vi "Open COM Port.vi"(8 "error in (no error)":errorcluster) -> (0 "error out":errorcluster, 3 "VISA Refnum out":refnum<visa-resource-name>)   [LabVIEW 2017]
uses:
  <vilib>/Instr/_visa.llb/VISA Configure Serial Port (Instr).vi
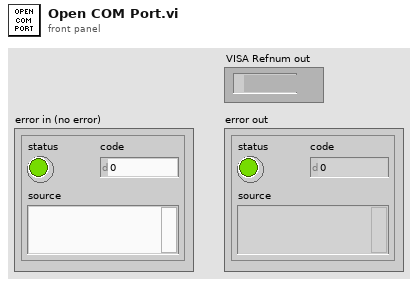
[diagram p1: front panel]
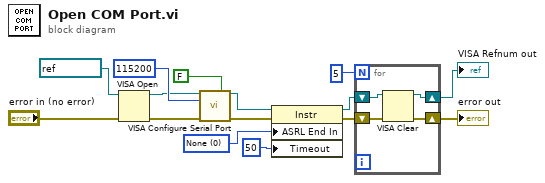
[diagram p0: block diagram]
diagram:
  w7 = u16 0 items=["None", "Last Bit", "TermChar"] ("Serial Settings:End Mode for Reads")
  n1 = VISA Open(error in (no error)="error in (no error)", VISA resource name=refnum<visa-resource-name> "COM2") -> (VISA resource name=w3:refnum<visa-resource-name>, error out=w2:errorcluster)  [unwired: 3 in]
  n2 = call-poly "VISA Configure Serial Port"("VISA resource name"=w3, "Enable Termination\nChar (T)"=FALSE ("Enable Termination\nChar (T)"), "baud rate (9600)"=u32 115200, "error in (no error)"=w2) -> ("VISA resource name out"=w6:refnum<visa-resource-name>, "error out"=w8:errorcluster)  [unwired: 10 in]
  n3 = property class="Instr"(reference=w6, error in=w8, "ASRL End In"=w7, "Timeout"=u32 50 ("General Settings:Timeout Value")) -> (reference out=w10:refnum<visa-resource-name>, error out=w11:errorcluster)
  n4 = for {
    N: 5 -> [_]
    shift-right: [w18] -> w15
    shift-left: w10 -> [w19]
    shift-right: [w17] -> w14
    shift-left: w11 -> [w16]
    n5 = VISA Clear(VISA resource name=w19, error in (no error)=w16) -> (VISA resource name out=w18:refnum<visa-resource-name>, error out=w17:errorcluster)
  }
  "VISA Refnum out" <- w15
  "error out" <- w14
